vi "Wait for ACK.vi"(8 "Error In":errorcluster, 11 "VISA in":refnum<visa-resource-name>) -> (0 "Error Out":errorcluster, 2 "ACK?":bool, 3 "VISA out":refnum<visa-resource-name>)   [LabVIEW 2014]
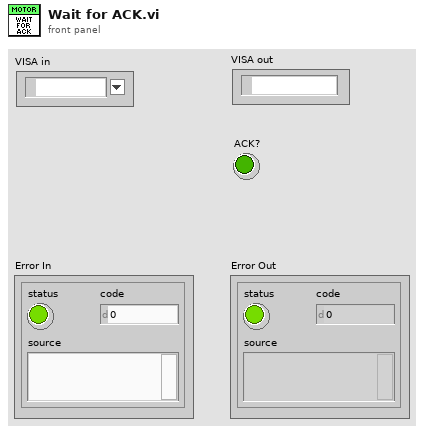
[diagram p1: front panel]
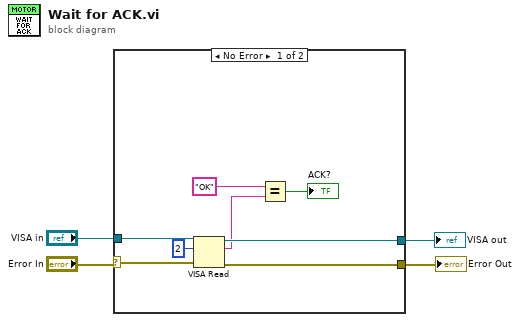
[diagram p0: block diagram]
diagram:
  n1 = case shown="No Error" "Error In" {
    selector: "Error In" -> [w11 w14]
    tunnel: "VISA in" -> [w12 w13]
    tunnel: [w9 w14] -> w1
    tunnel: [w8 w13] -> w2
    frame No Error {
      n2 = VISA Read(VISA resource name=w12, byte count=u32 2, error in (no error)=w11) -> (VISA resource name out=w8:refnum<visa-resource-name>, read buffer=w7:string, error out=w9:errorcluster)  [unwired: 1 out]
      n3 = Equal?(x="OK", y=w7) -> (x = y?=→"ACK?":bool)
    }
    frame Error {
    }
  }
  "VISA out" <- w2
  "Error Out" <- w1
